vi "AlliGator Decay Graph Get-Set Process Plot Target.vi"(6 "Get (F)/Set":bool, 8 "Error In":errorcluster, 9 "Plot(s) to Process":T1, 11 "Menu":refnum<k9>) -> (0 "Error Out (dup)":errorcluster, 1 "Plot(s) to Process":T1, 3 "Menu":refnum<k9>)   [LabVIEW 2021, in "AlliGator Decay Analysis.lvlib" / "AlliGator Decay Processing.lvlib"]
doc: "<B>Get</B>: Check which plot(s) to process, and add/remove checkmarks accordingly. In this case, the <B>Menu</B> reference is mandatory.\n\n<B>Set</B>: based on user selection, set which plot(s) to process. In this case, the <B>Plot(s) to Process</B>input is mandatory (Single Plot, Selected Plots, All Plots), but not the <B>Menu</B>."
uses:
  AlliGator Decay Processing.lvlib
  AlliGator Decay Graph Process Plot Target.ctl
  AlliGator Variables List.ctl
  AlliGator Globals, Variables & Constants.lvlib
  AlliGator Decay Analysis.lvlib
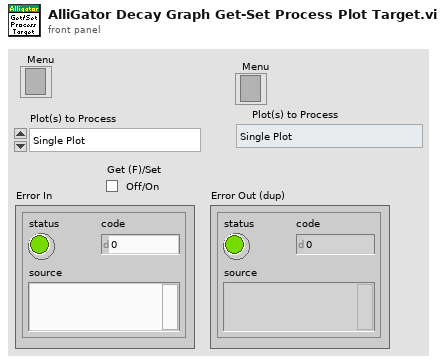
[diagram p1: front panel]
types:
  T1 = typedef "AlliGator Decay Analysis.lvlib/AlliGator Decay Graph Process Plot Target.ctl" = enum16{"Single Plot", "Selected Plots", "All Plots"}
  T2 = typedef "AlliGator Globals, Variables & Constants.lvlib/AlliGator Variables List.ctl" = enum16{"---- GUI ----", "Initialization Status", "State Indicators Refnum", "Original AlliGator Menu Items", "Current Action Loop State", "Script in progress", "Playback", "Loop Playback", "Search ROI Used", "Search ROI", "Decay Graph Max Legend Size", "Intensity Graph Max Legend Size", "Decay Statistics Graph Max Legend Size", "Phasor Graph Max Legend Size", "Phasor Ratio Graph Max Legend Size", "Lifetime Graph Max Legend Size", "---- Files ----", "Export Dataset Frames as Individual Files", "Show Batch Export Help Balloons", "Frames in Dataset", "ptu File Frame Start Indices", "Current Frame in Dataset", "Current Frame Timestamp", "------ Python Plugins ------", "Python Plugins Information", "Python Session", "Valid Python Session?", "---- Source Image ----", "Dataset Loaded", "Dataset Metadata", "Dataset Channel", "Dataset Data Description", "Background Dataset Metadata", "Background Dataset Channel", "Background Dataset Data Description", "Background File Subtraction", "Background File Path", "Background File Pile-up Correction", "Background File Pixel Well Capacity", "Background File Scaling Factor", "Source Image ROIs", "Current Source Image ROI", "Source Image ROI Event Refnum", "X_Source Image Display Range", "X_Source Image Palette Information", "Source Image Palette List", "Source Image Scale", "Current Dataset Load Settings", "Source Image:ROI Overlay Color", "---- Image Profile Window ----", "Image Profile:Overlay ROI in Source Image", "Image Profile Window Event Refnum", "Image Profile:IntensityType", "Image Profile:Intensity Average Type", "Image Profile:Intensity-weighted SDV", "Image Profile:Box Profile Type", "Image Profile Window Open", "Image Profile:Plotted Fit Parameter", "X_Type of Displayed Image", "X_Time Gate Slider", "Dataset Path", "Source Image Overlay to Erase", "Is Displayed Image Accumulated", "White Light Image Modified", "Mask Image Modified", "Macrotime Gate Separation", "------ Phasor Graph -------", "Phasor Graph:Show Line", "---- Phasor Plot ---", "Phasor Plot Parameters Changed", "FLI Dataset Modified since last Phasor Plot Calculation", "Phasor Harmonics Data", "Selected Phasor Harmonics", "Phasor Harmonic Manager Event Refnum", "Phasor Plot ROIs", "Current Phasor Plot ROI", "Phasor Plot ROI Event Refnum", "Phasor Plot Image Reference Points", "Phasor Plot Computed", "Phasor Plot Palette Information", "Phasor Plot Palette List", "Phasor Ratio Palette Information", "Phasor Ratio Palette List", "Phasor Image Scale", "Phasor Plot Image Overlay to Erase", "Phasor Plot Image Elements to Update", "Current Phasor Plot Calculation Parameters", "Current Phasor Calibration Options", "Reset Cumulated Phasor Plot", "Phasor Ratio Reference 1", "Phasor Ratio Lifetime Reference 1", "Phasor Ratio Reference 1 Frequency", "Phasor Ratio Reference 2", "Phasor Ratio Lifetime Reference 2", "Phasor Ratio Reference 2 Frequency", "---- Decay Analysis ----", "Number of Selected Decays to Fit", "LS Fit Results", "LAR Fit Results", "BS Fit Results", "Last Decay Max - Min", "Best Fit Parameters", "Best Fit Parameter Names", "Actual Size X", "Actual Size Y", "Binning X", "Binning Y", "Actual # Gates", "Dataset Number", "Gates to...", "Gates Skipped", "Gates to keep", "Gate Step", "Gate Separation", "Reversed Gates", "Pile-up Correction", "Pixel Well Capacity", "Background Subtracted", "Background Subtraction Method", "Background Definition Range", "Background File (deprecated)", "Number of Dataset Accumulated", "Array of Accumulated Dataset Paths", "Do Averaged Datasets", "Destination File Path", "Process Plot Target", "Use 1/D as Phasor Frequency", "---- Decay Fit Parameter Map -----", "Decay Fit Parameter Map Palette Information", "Decay Fit Parameter Map Palette List", "Local Decay Graph Window Event Refnum", "------- Local Decay Window ---------", "Use normalized IRF for convolution", "----- Miscellaneous ----", "Skippable Dialog Windows Status"}
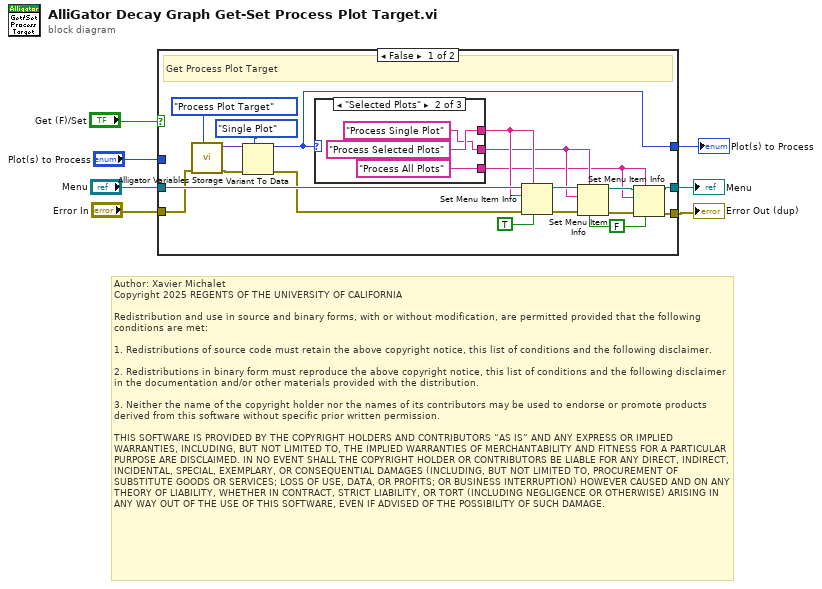
[diagram p0: block diagram]
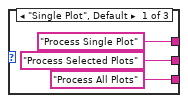
[diagram p2: hidden frame]
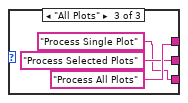
[diagram p3: hidden frame]
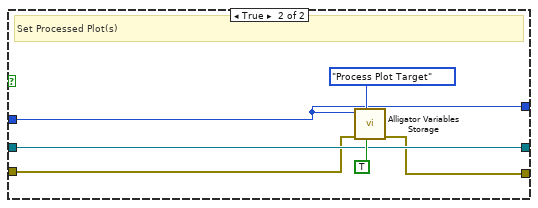
[diagram p4: hidden frame]
diagram:
  # "Author: Xavier Michalet\nCopyright 2025 REGENTS OF THE UNIVERSITY OF CALIFORNIA\n\nRedistribution and use in source and binary forms, with or without modification, are permitted provided that the following conditions are met:\n\n1. Redistributions of source code must retain the above copyright notice, this list of conditions and the following disclaimer.\n\n2. Redistributions in binary form must reproduce the above copyright notice, this list of conditions and the following disclaimer in the documentation and/or other materials provided with the distribution.\n\n3. Neither the name of the copyright holder nor the names of its contributors may be used to endorse or promote products derived from this software without specific prior written permission.\n\nTHIS SOFTWARE IS PROVIDED BY THE COPYRIGHT HOLDERS AND CONTRIBUTORS “AS IS” AND ANY EXPRESS OR IMPLIED WARRANTIES, INCLUDING, BUT NOT LIMITED TO, THE IMPLIED WARRANTIES OF MERCHANTABILITY AND FITNESS FOR A PARTICULAR PURPOSE ARE DISCLAIMED. IN NO EVENT SHALL THE COPYRIGHT HOLDER OR CONTRIBUTORS BE LIABLE FOR ANY DIRECT, INDIRECT, INCIDENTAL, SPECIAL, EXEMPLARY, OR CONSEQUENTIAL DAMAGES (INCLUDING, BUT NOT LIMITED TO, PROCUREMENT OF SUBSTITUTE GOODS OR SERVICES; LOSS OF USE, DATA, OR PROFITS; OR BUSINESS INTERRUPTION) HOWEVER CAUSED AND ON ANY THEORY OF LIABILITY, WHETHER IN CONTRACT, STRICT LIABILITY, OR TORT (INCLUDING NEGLIGENCE OR OTHERWISE) ARISING IN ANY WAY OUT OF THE USE OF THIS SOFTWARE, EVEN IF ADVISED OF THE POSSIBILITY OF SUCH DAMAGE."
  n1 = case shown="False" "Get (F)/Set" {
    tunnel: "Menu" -> [w26 w39]
    tunnel: "Error In" -> [w25 w38]
    tunnel: [w24 w37] -> w5
    tunnel: [w23 w39] -> w4
    tunnel: "Plot(s) to Process" -> [_ w36]
    tunnel: [w8 w36] -> w1
    frame False {
      w10 = FALSE ("checked")
      # "Get Process Plot Target"
      n2 = call "Alligator Variables Storage.vi"("AlliGator Variable"=AlliGator_Variables_List."Process Plot Target" ("Alligator Variable"), "Error In"=w25) -> ("Error Out"=w20:errorcluster, "Data out"=w21:variant)  [unwired: 7 in, 1 out]
      n3 = Variant To Data(error in=w20, type=AlliGator_Decay_Graph_Process_Plot_Target."Single Plot" ("Process Plot Target"), Variant=w21) -> (data=w8:T1, error out=w19:errorcluster)
      n4 = case shown="\"Selected Plots\"" w8 {
        tunnel: ["Process Single Plot" ("item tag") "Process Selected Plots" ("item tag") "Process All Plots" ("item tag")] -> w15
        tunnel: ["Process Selected Plots" ("item tag") "Process Single Plot" ("item tag") "Process Selected Plots" ("item tag")] -> w14
        tunnel: ["Process All Plots" ("item tag") "Process All Plots" ("item tag") "Process Single Plot" ("item tag")] -> w12
        frame "Single Plot", Default {
        }
        frame "Selected Plots" {
        }
        frame "All Plots" {
        }
      }
      n5 = Set Menu Item Info(6:TRUE ("checked"), 7:w15, 8:w19, 10:w15, 11:w26) -> (0:w16:errorcluster, 3:w17:refnum<k9>)  [unwired: 2 in]
      n6 = Set Menu Item Info(6:w10, 7:w14, 8:w16, 10:w14, 11:w17) -> (0:w11:errorcluster, 3:w13:refnum<k9>)  [unwired: 2 in]
      n7 = Set Menu Item Info(6:w10, 7:w12, 8:w11, 10:w12, 11:w13) -> (0:w24:errorcluster, 3:w23:refnum<k9>)  [unwired: 2 in]
    }
    frame True {
      # "Set Processed Plot(s)"
      n8 = call "Alligator Variables Storage.vi"("Get(F)/Set"=TRUE, "AlliGator Variable"=AlliGator_Variables_List."Process Plot Target" ("Alligator Variable"), "Error In"=w38, "Data in"=w36) -> ("Error Out"=w37:errorcluster)  [unwired: 5 in, 2 out]
    }
  }
  "Error Out (dup)" <- w5
  "Menu" <- w4
  "Plot(s) to Process" <- w1
